vi "Navigation_Main_position_testing may 2.vi"() -> ()   [LabVIEW 2015]
uses:
  <vilib>/myRIO/Instrument Drivers/Onboard IO/PWM/typedefs/PWM Reference.ctl
  <vilib>/myRIO/Common/Instrument Driver Framework/Utilities/typedefs/myRIO Generic Hardware Reference.ctl
  <vilib>/myRIO/Common/Instrument Driver Framework/Utilities/typedefs/Hardware Version Enum.ctl
  <vilib>/myRIO/Common/Instrument Driver Framework/Utilities/typedefs/myRIO v1.0 Reference.ctl
  <vilib>/myRIO/Common/Instrument Driver Framework/Utilities/typedefs/Generic FPGA Reference.ctl
  <vilib>/myRIO/Common/Instrument Driver Framework/myRIO v1.0/PWM/typedefs/PWM Channels Enum.ctl
  <vilib>/myRIO/Instrument Drivers/Onboard IO/PWM/typedefs/PWM Configuration.ctl
  <vilib>/userdefined/High Color/nirio_resource_hc.ctl
  <vilib>/myRIO/Common/Instrument Driver Framework/myRIO v1.0/PWM/vis/myRIO v1.1 Open PWM.vi
  <vilib>/myRIO/Common/Instrument Driver Framework/Utilities/vis/Validate Channels.vi
  <vilib>/myRIO/Common/Instrument Driver Framework/myRIO v1.0/PWM/vis/myRIO v1.0 Reserve PWM.vi
  <vilib>/myRIO/Common/Instrument Driver Framework/myRIO v1.0/PWM/vis/myRIO v1.0 Build MUX Configuration PWM.vi
  <vilib>/myRIO/Common/Instrument Driver Framework/myRIO v1.0/Resource Manager/vis/myRIO v1.0 Reserve Channel List.vi
  <vilib>/myRIO/Common/Instrument Driver Framework/myRIO v1.0/Resource Manager/vis/myRIO v1.0 Create Configuration List.vi
  <vilib>/myRIO/Common/Instrument Driver Framework/myRIO v1.0/Resource Manager/vis/myRIO v1.0 Reserve Channel.vi
  <vilib>/myRIO/Common/Instrument Driver Framework/myRIO v1.0/Resource Manager/vis/myRIO v1.0 Unreserve Channel.vi
  <vilib>/myRIO/Common/Instrument Driver Framework/myRIO v1.0/Resource Manager/vis/myRIO v1.0 Build Mutex Name.vi
  <vilib>/FPGAPlugInAG/myRIO-1900/niLvFpga_Open_myRIO-1900.vi
  <vilib>/rvi/interface/common/dynamic/niFpgaDynamicAddResources.vi
  <vilib>/myRIO/Common/Instrument Driver Framework/Utilities/vis/FPGA Ref Manager.vi
  <vilib>/Utility/error.llb/Error Cluster From Error Code.vi
  <vilib>/myRIO/Common/Instrument Driver Framework/Utilities/vis/Ref Counter.vi
  <vilib>/rvi/errors/niLvFpgaAdjustHostInterfaceError.vi
  <vilib>/Utility/VariantDataType/GetNumericInfo.vi
  <vilib>/myRIO/Common/Instrument Driver Framework/myRIO v1.0/myRIO v1.1 Open.vi
  <vilib>/myRIO/Common/Instrument Driver Framework/Utilities/vis/IO Manager.vi
  <vilib>/myRIO/Common/Instrument Driver Framework/Utilities/vis/Configuration Manager.vi
  <vilib>/myRIO/Common/Instrument Driver Framework/myRIO v1.0/Resource Manager/vis/myRIO v1.0 Configure IO.vi
  <vilib>/myRIO/Common/Instrument Driver Framework/myRIO v1.0/myRIO v1.0 Close.vi
  <vilib>/myRIO/Common/Instrument Driver Framework/myRIO v1.0/PWM/vis/myRIO v1.0 Write PWM.vi
  <vilib>/addons/control/pid/pid.llb/PID (DBL).vi
  <vilib>/rvi/interface/nirviOpenFPGA/nirviOpenFPGA.xnode
  Navi/E/FPGA Bitfiles/NavigationProjec_FPGATarget2_FPGAMainNavigati_PWPHW8gwDxI.lvbitx
  <vilib>/rvi/interface/nirviReadWriteControl/nirviReadWriteControl.xnode
  <vilib>/myRIO/Instrument Drivers/Onboard IO/PWM/vis/myRIO PWM Open.xnode
  <vilib>/myRIO/Instrument Drivers/Onboard IO/PWM/PWM.lvlib
  <vilib>/myRIO/Instrument Drivers/Utilities/Utilities.lvlib
  NiFpgaLv.dll
  <vilib>/rvi/interface/Simulation/niFpgaSimulationCallBeginRW.vi
  <vilib>/addons/control/pid/NI_PID_pid.lvlib
panel:
  out "y1ahead":dbl
  out "angle error":dbl
  out "percent away from x goal":dbl
  out "y desired":dbl
  out "slope desired":dbl
  out "orientation theta desired":dbl
  out "current angle":dbl
  out "current y":dbl
  out "current x":dbl
  out "mining angle":dbl
  out "mining y":dbl
  out "mining x":dbl
  out "mining location":dbl=1.0
  out "distance to goal":dbl
  out "loc_y":dbl
  out "loc_x":dbl
  out "loc_theta":dbl
  in  "motor killswitch":bool
  in  "set start position":bool
  in  "dumping complete":bool
  in  "digging complete?":bool
  in  "position good?":bool
  in  "state":dbl
  in  "case":dbl
  in  "x goal":dbl=9.0
  in  "Encoder Reset":bool
  out "scale":dbl=1.0
  out "reset x y 2":dbl
  out "stop motors":dbl
  out "encoder stop switch":dbl=1.0
  out "left wheels actual pwm":dbl
  out "right wheels actual pwm":dbl
  out "desired pwm right":dbl
  out "desired pwm left":dbl
  out "left setpoint":dbl
  out "right setpoint":dbl
  in  "PID Settings":enum32{"Right PID PWM", "Left PID PWM"}(tab)
  in  "output range right":cluster{"output high":dbl, "output low":dbl}={"output high"=0.13333, "output low"=-0.13333} {"output low" format="%.6f"; "output high" format="%.5f"}
  in  "PID gains right":T1={"proportional gain (Kc)"=0.002, "integral time (Ti, min)"=7e-07, "derivative time (Td, min)"=0.0} {"derivative time (Td, min)" format="%.8f"; "integral time (Ti, min)" format="%.8f"; "proportional gain (Kc)" format="%.8f"}
  out "dt out (s) right":dbl format="%.3f"
  out "PID feedback Right":dbl
  out "Elapsed Time (s) Right":dbl caption="Elapsed Time (s)"
  in  "pid reset right":bool
  in  "output range left":cluster{"output high":dbl, "output low":dbl}={"output high"=0.13333, "output low"=-0.13333} {"output low" format="%.6f"; "output high" format="%.5f"}
  in  "PID gains left":T1={"proportional gain (Kc)"=0.002, "integral time (Ti, min)"=7e-07, "derivative time (Td, min)"=0.0} {"derivative time (Td, min)" format="%.8f"; "integral time (Ti, min)" format="%.8f"; "proportional gain (Kc)" format="%.8f"}
  out "dt out (s) left":dbl format="%.3f"
  out "PID feedback Left":dbl
  out "Elapsed Time (s) Left":dbl caption="Elapsed Time (s)"
  in  "pid reset left":bool
  out "start angle":dbl=1.0
  out "start x":dbl=1.0
  out "start y":dbl
  in  "stuff that i dont want to mess with right now":T2(tab)
  out "RM Linear Velocity (rot/s)":dbl
  out "RR Rot Velocity (rot/s)":dbl
  out "LR Rot Velocity (rot/s)":dbl
  out "LM Rot Velocity (rot/s)":dbl
  out "LF Rot Velocity (rot/s)":dbl
  out "RF Linear Velocity (rot/s)":dbl
  out "Tick Count(mSec) 2":u32 caption="Tick Count(mSec)"
  out "y traveled 2":dbl
  out "x traveled 2":dbl
  out "y position 2":dbl
  out "x position 2":dbl
  out "y dot 2":dbl
  out "distance traveled 2":dbl
  out "psi dot 2":dbl
  out "x dot 2":dbl
  out ".not. x? 2":bool
  out ".not. x? 3":bool
  out "goal reached":bool=TRUE
  out "avg ENC.B":dbl
  out "avg ENC.A":dbl
  out "ENC.B_c.CNTR":i32
  out "ENC.B_b.CNTR":i32
  out "ENC.B_a.CNTR":i32
  out "ENC.A_c.CNTR":i32
  out "ENC.A_b.CNTR":i32
  out "ENC.A_a.CNTR":i32
  out "stage set point parameters":T3(tab)
  out "x straight 1 end":dbl=2.0
  in  "ypstart straight 1":dbl
  in  "ystart":dbl=1.0
  in  "yend straight 1":dbl=2.0
  in  "ypend straight 1":dbl
  out "a straight 1":dbl
  out "b straight 1":dbl
  out "c straight 1":dbl
  out "d straight 1":dbl
  out "x turn end":dbl=7.0
  in  "ystart turn":dbl=1.0
  in  "yend turn":dbl=2.0
  in  "ypstart turn":dbl
  in  "ypend turn":dbl
  out "a turn":dbl
  out "b turn":dbl
  out "c turn":dbl
  out "d turn":dbl
  out "x straight 2 end":dbl=10.0
  in  "yend straight 2":dbl=2.0
  out "a straight 2":dbl
  out "b straight 2":dbl
  out "c straight 2":dbl
  out "d straight 2":dbl
  in  "ypend 2":dbl
  in  "ypstart straight 2":dbl
  in  "mining y 1":dbl=2.0
  in  "mining angle 1":dbl
  in  "mining x 1":dbl=9.0
  in  "mining angle -1":dbl
  in  "mining y -1":dbl=4.0
  in  "mining x -1":dbl=9.0
  out "left pwm":dbl(graph)
  out "right pwm":dbl(graph)
  out "SYS.SELECTA":u8 format="%08b"
  in  "R Min Linear Velocity (ft/s)":dbl=-2.0 format="%#_13g"
  in  "R Max Linear Velocity (ft/s)":dbl=2.0 format="%#_13g"
  in  "L Min Linear Velocity (ft/s)":dbl=-2.0 format="%#_13g"
  in  "L Max Linear Velocity (ft/s)":dbl=2.0 format="%#_13g"
  out "Current Rot Velocity (rot/s)":T4(graph)
  # "Position Information"
  # "move cases along"
  # "end state 0\ngo to state 1"
  # "end state 1\ngo to state 2"
  # "end state 2\ngo to state 3"
  # "end state 3\ngo to state 4"
  # "end state 4\ngo to state 0"
  # "same thing, redundant \nbut can be changed to \nsomething useful later"
  # "this must be true to \ninitialize the routine"
  # "go through the 3\n movement cases"
  # "go through the 3\n movement cases"
  # "Stop Flags \n1=go \n0=stop"
  # "PWM Setpoint"
  # "Initial condtions"
  # "Encoder Values"
  # "Motor Control Parameters"
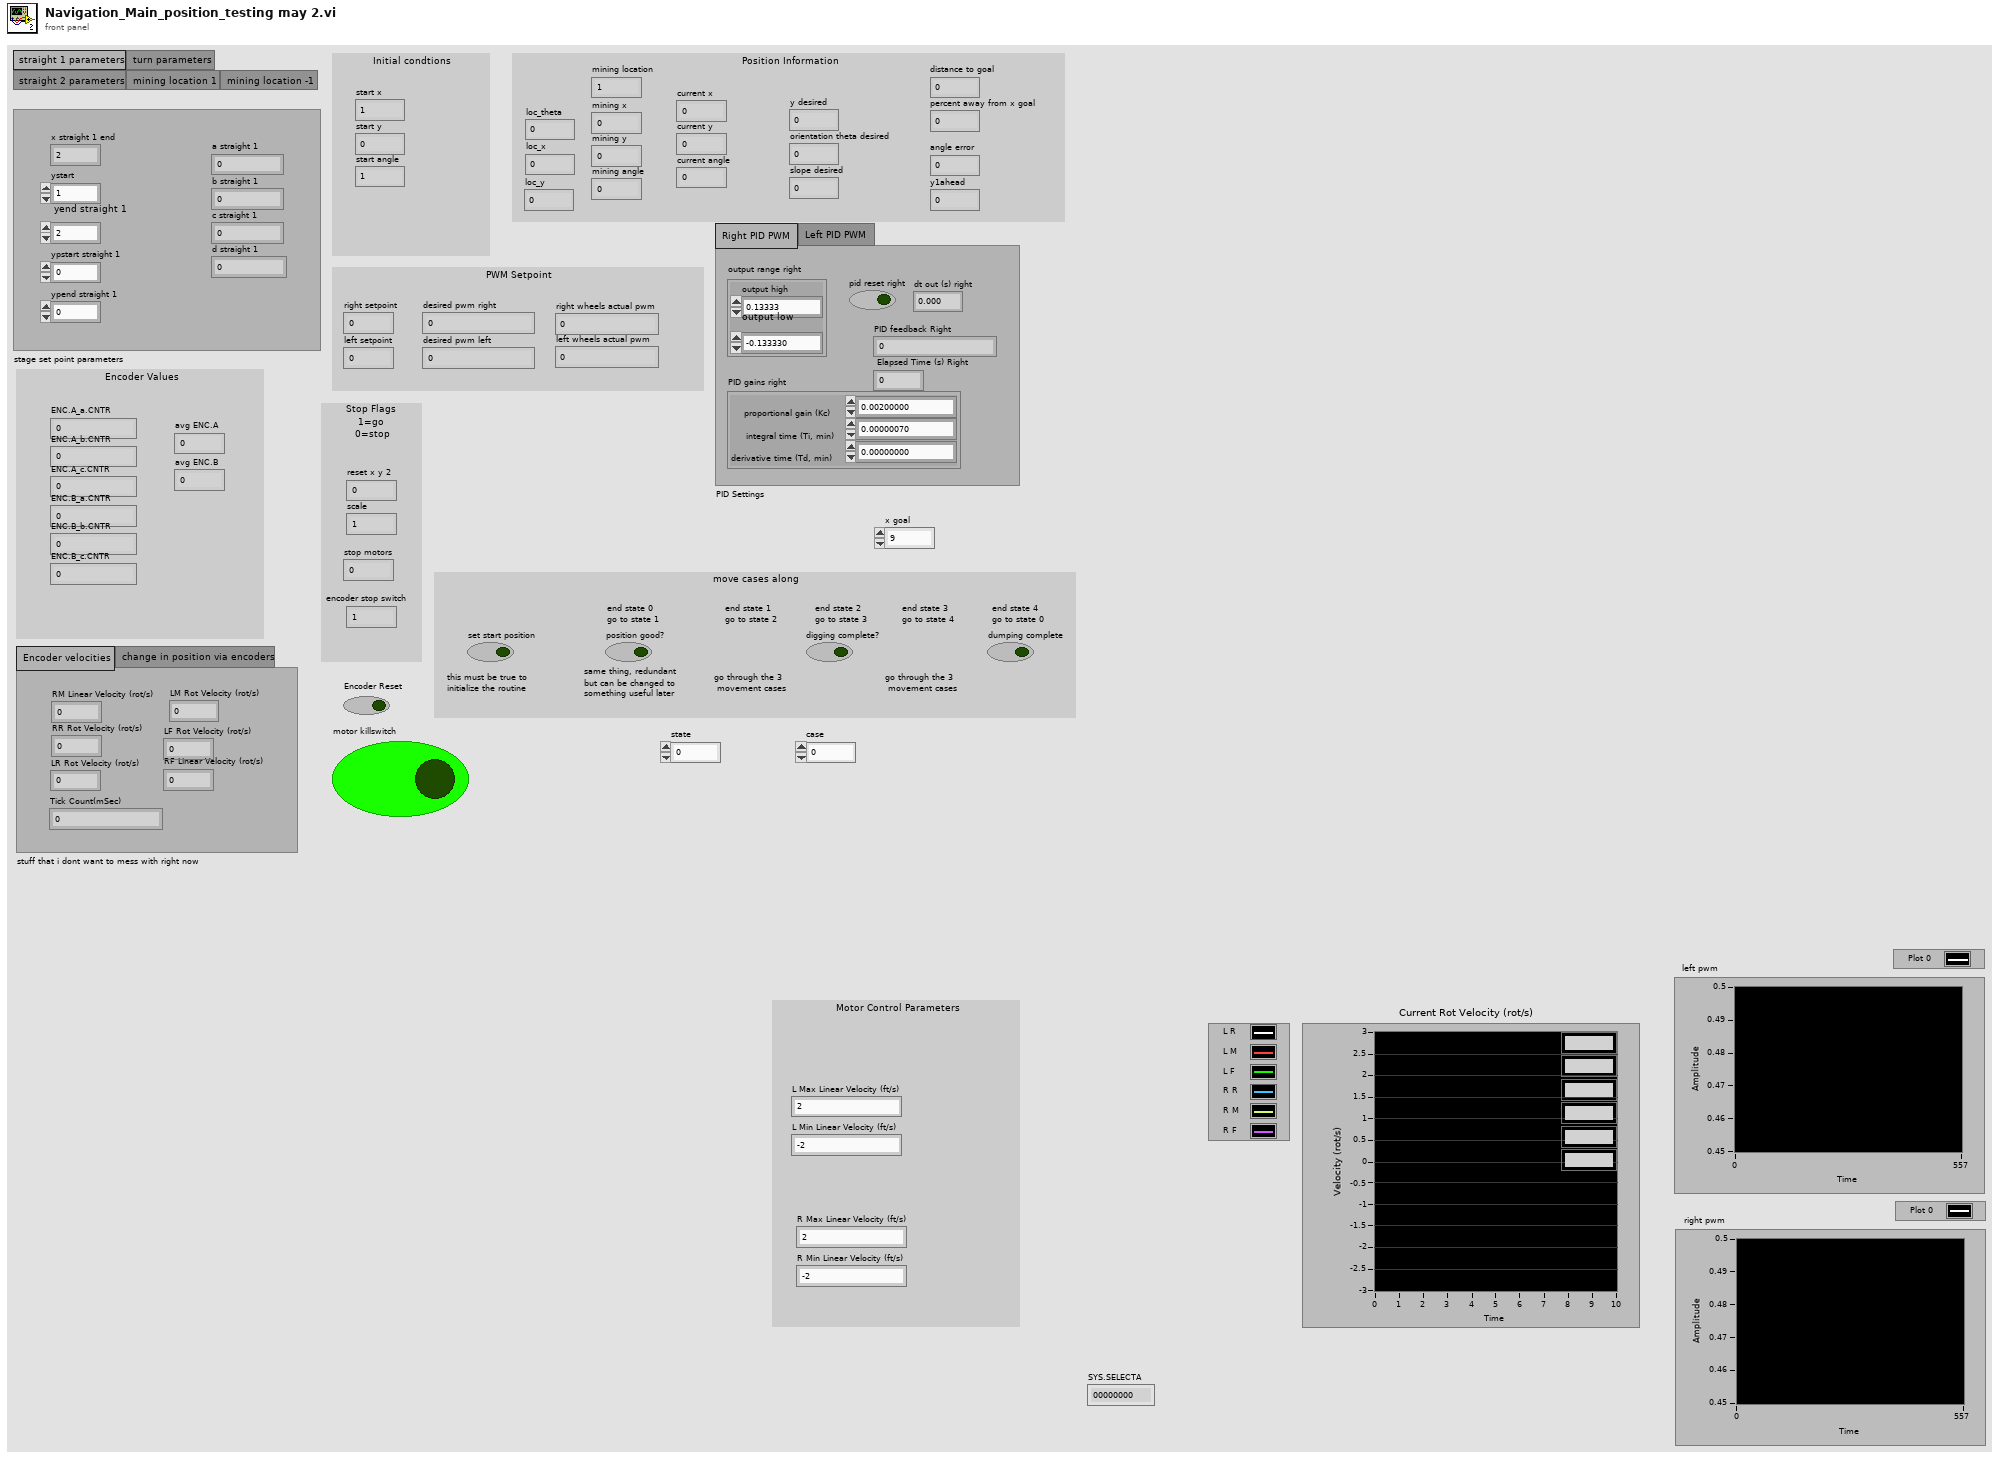
[diagram p1: front panel]
types:
  T1 = cluster{"proportional gain (Kc)":dbl, "integral time (Ti, min)":dbl, "derivative time (Td, min)":dbl}
  T2 = enum32{"Encoder velocities", "change in position via encoders"}
  T3 = enum32{"straight 1 parameters", "turn parameters", "straight 2 parameters", "mining location 1", "mining location -1"}
  T4 = cluster{"Rotational Velocity (RPS)":dbl, "Rotational Velocity (RPS)":dbl, "Rotational Velocity (RPS)":dbl, "Rotational Velocity (RPS)":dbl, "Rotational Velocity (RPS)":dbl, "Rotational Velocity (RPS)":dbl}
  T5 = typedef "nirio_resource_hc.ctl" = tag
  T6 = typedef "Hardware Version Enum.ctl" = enum16{"Unknown", "myRIO-1900", "myRIO-1950", "roboRIO"}
  T7 = typedef "PWM.lvlib/PWM Reference.ctl" = cluster{"myRIO Reference":T8, "PWM Channels Enum":T11, "PWM Configuration":T12}
  T8 = typedef "myRIO Generic Hardware Reference.ctl" = cluster{"myRIO Model":T6, "myRIO Hardware Reference":T9}
  T9 = typedef "myRIO v1.0 Reference.ctl" = cluster{"Generic FPGA Reference":T10, "Allow multiple opens":bool}
  T10 = typedef "Generic FPGA Reference.ctl" = refnum<k20>
  T11 = typedef "PWM Channels Enum.ctl" = enum16{"Not Connected", "C/PWM0", "C/PWM1", "A/PWM0", "A/PWM1", "A/PWM2", "B/PWM0", "B/PWM1", "B/PWM2", "PWM/PWM0", "PWM/PWM1", "PWM/PWM2", "PWM/PWM3", "PWM/PWM4", "PWM/PWM5", "PWM/PWM6", "PWM/PWM7", "PWM/PWM8", "PWM/PWM9"}
  T12 = typedef "PWM.lvlib/PWM Configuration.ctl" = cluster{"Frequency":dbl, "Duty Cycle":dbl}
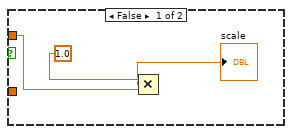
[diagram p3: hidden frame]
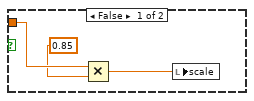
[diagram p4: hidden frame]
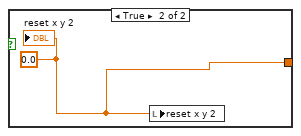
[diagram p5: hidden frame]
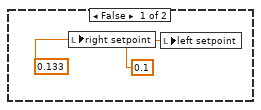
[diagram p6: hidden frame]
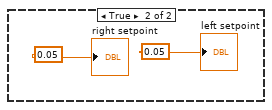
[diagram p7: hidden frame]
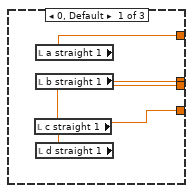
[diagram p8: hidden frame]
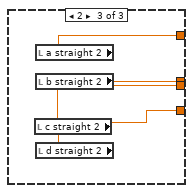
[diagram p9: hidden frame]
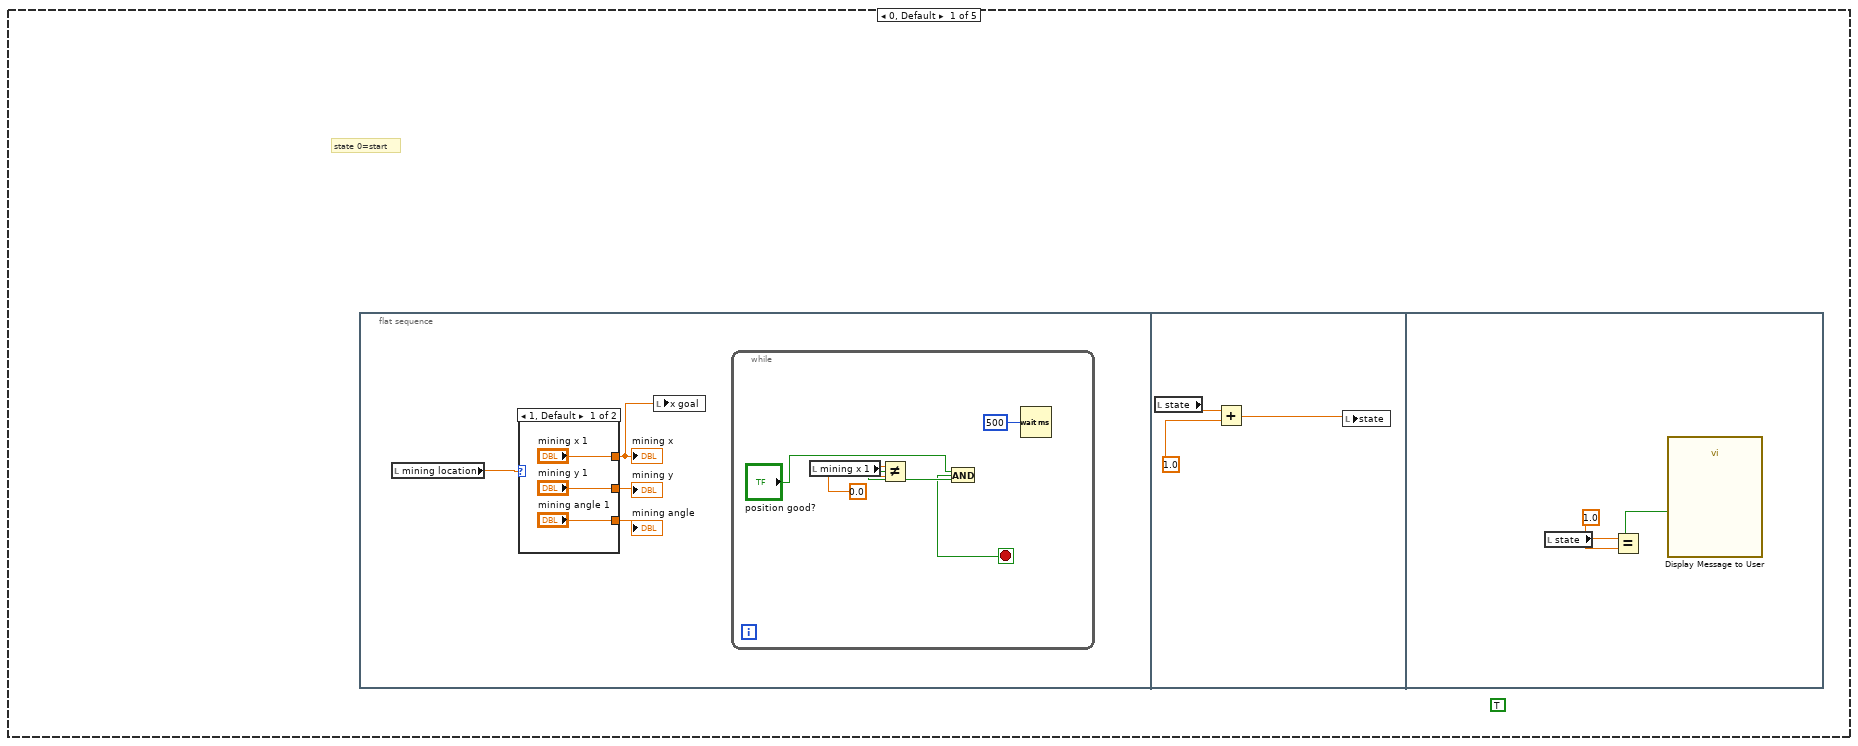
[diagram p10: hidden frame]
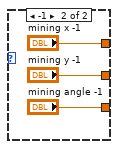
[diagram p11: hidden frame]
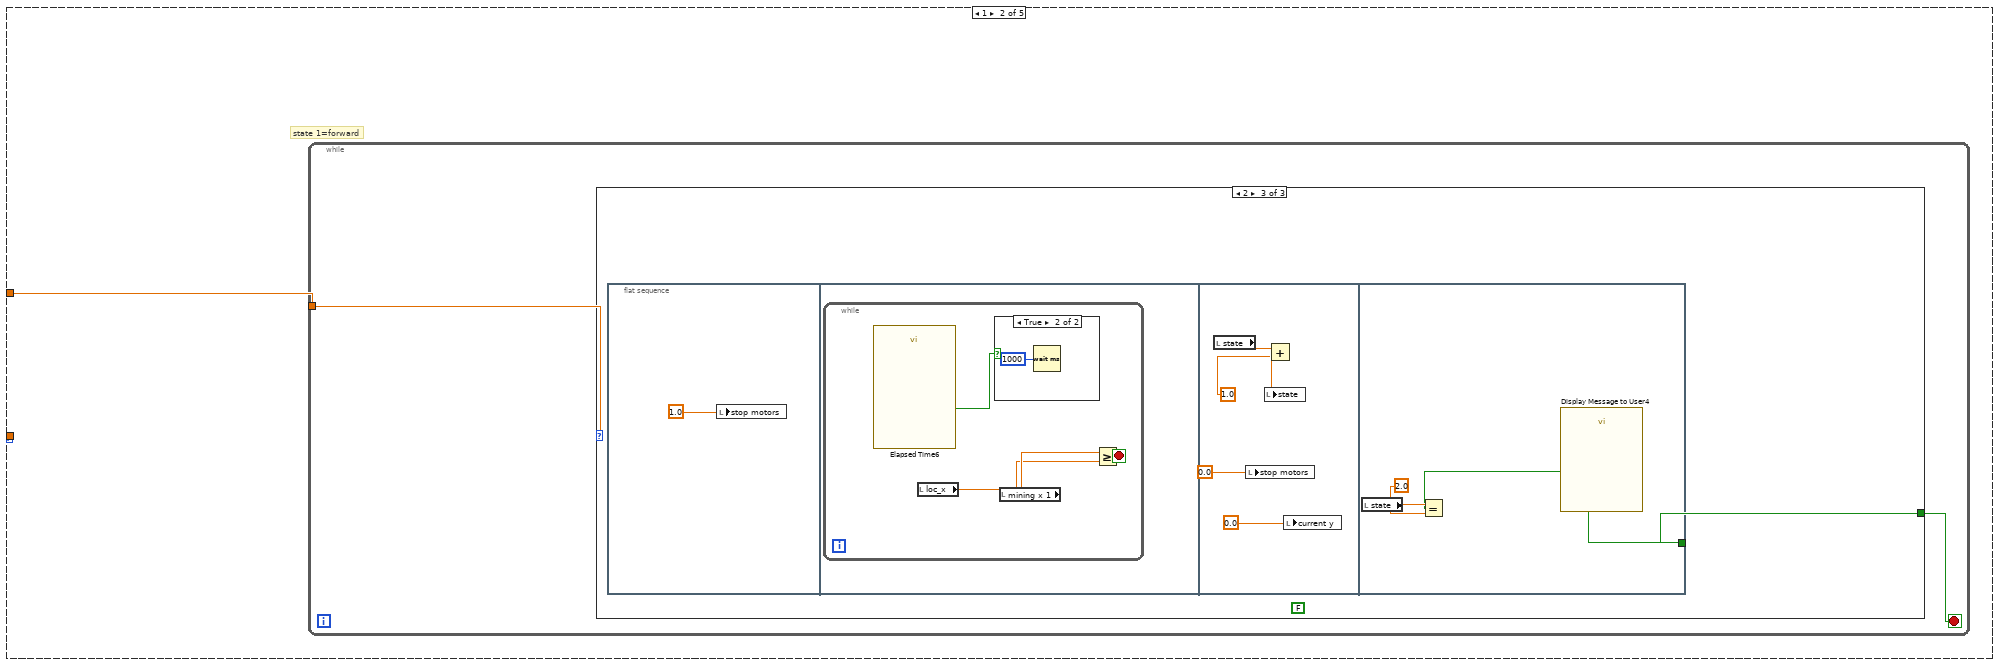
[diagram p12: hidden frame]
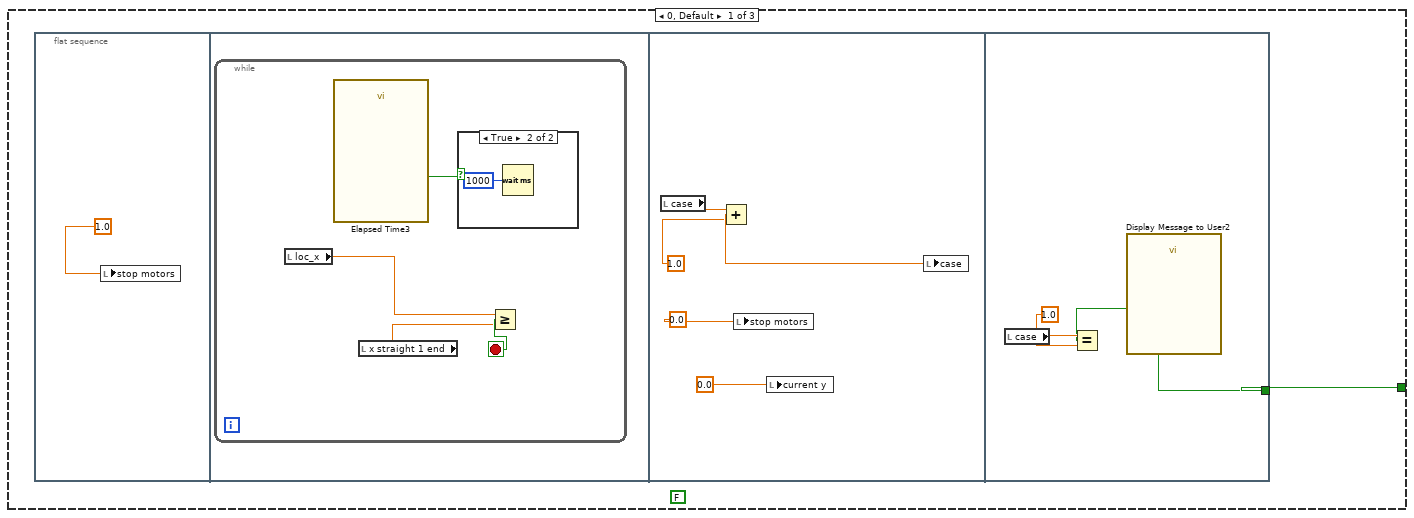
[diagram p13: hidden frame]
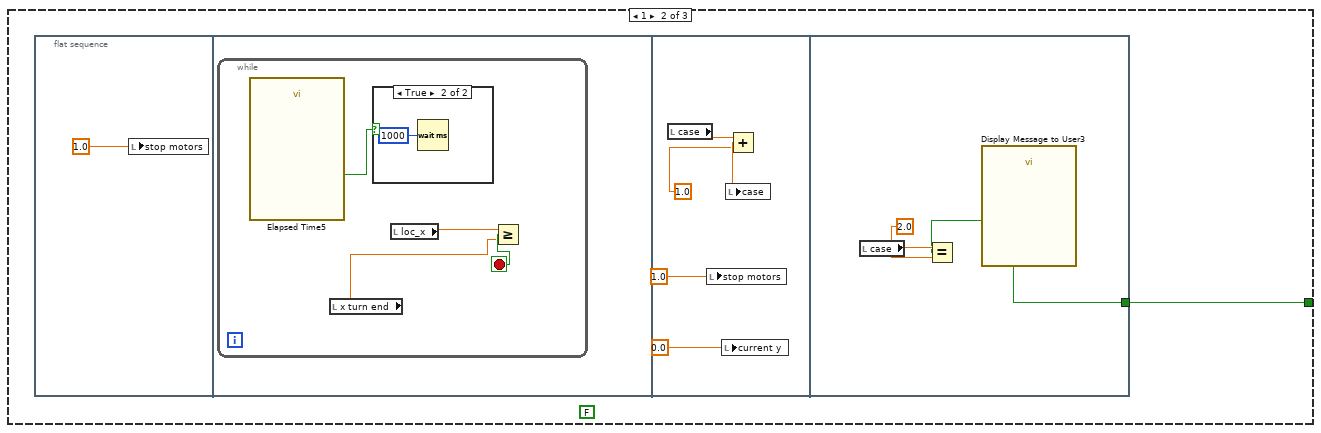
[diagram p15: hidden frame]
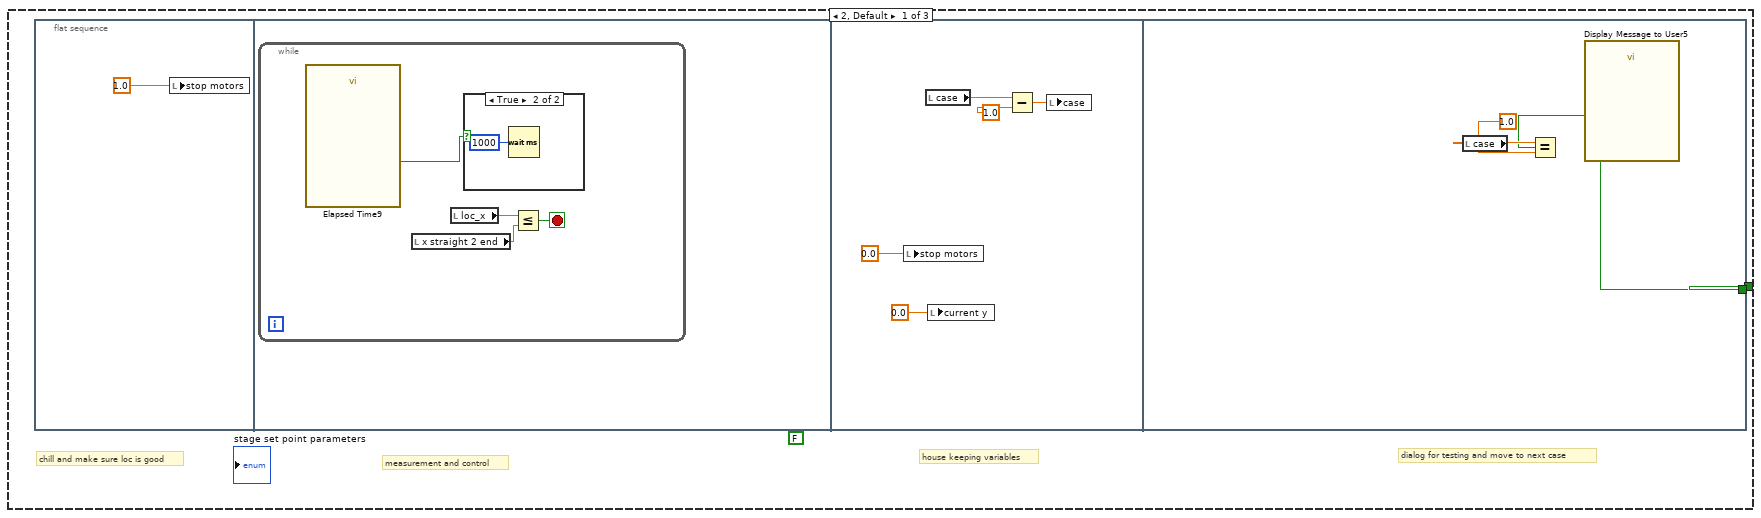
[diagram p18: hidden frame]
diagram:
  n1 = flat-sequence {
    tunnel: [w33] -> w30
    tunnel: [w33] -> w29
    tunnel: [w46] -> w28
    tunnel: [w61] -> w26
    tunnel: [w57] -> w24
    tunnel: [w56] -> w22
    tunnel: [w55] -> w20
    tunnel: [w54] -> w18
    tunnel: [w53] -> w16
    tunnel: ["L Max Linear Velocity (ft/s)"] -> w14
    tunnel: ["L Min Linear Velocity (ft/s)"] -> w12
    tunnel: ["R Max Linear Velocity (ft/s)"] -> w10
    tunnel: ["R Min Linear Velocity (ft/s)"] -> w8
    tunnel: [w48] -> w6
    tunnel: w30 -> [w47]
    tunnel: [w47] -> w4
    tunnel: w29 -> [w48]
    tunnel: [w46] -> w2
    tunnel: w28 -> [w187]
    tunnel: [w187] -> w27
    tunnel: w26 -> [w186]
    tunnel: [w186] -> w25
    tunnel: w24 -> [w185]
    tunnel: [w185] -> w23
    tunnel: w22 -> [w184]
    tunnel: [w184] -> w21
    tunnel: w20 -> [w183]
    tunnel: [w183] -> w19
    tunnel: w18 -> [w182]
    tunnel: [w182] -> w17
    tunnel: w16 -> [w181]
    tunnel: [w181] -> w15
    tunnel: w14 -> [w180]
    tunnel: [w180] -> w13
    tunnel: w12 -> [w179]
    tunnel: [w179] -> w11
    tunnel: w10 -> [w178]
    tunnel: [w178] -> w9
    tunnel: w8 -> [w177]
    tunnel: [w177] -> w7
    tunnel: w6 -> [w176]
    tunnel: [w176] -> w5
    tunnel: w4 -> [w175]
    tunnel: [w175] -> w3
    tunnel: w2 -> [w174]
    tunnel: [w174] -> w1
    tunnel: w27 -> [_]
    tunnel: w25 -> [w196]
    tunnel: w23 -> [w202]
    tunnel: w21 -> [w199]
    tunnel: w19 -> [w198]
    tunnel: w17 -> [w197]
    tunnel: w15 -> [w201]
    tunnel: w13 -> [_]
    tunnel: w11 -> [_]
    tunnel: w9 -> [_]
    tunnel: w7 -> [_]
    tunnel: w5 -> [w204]
    tunnel: w3 -> [w203]
    tunnel: w1 -> [w200]
    frame #0 {
      n2 = flat-sequence {
        tunnel: w34 -> [w39]
        tunnel: [w37] -> w36
        tunnel: w36 -> [w41]
        tunnel: [w41] -> w35
        tunnel: w35 -> [w44]
        tunnel: [w43] -> w33
        frame #0 {
          w38 = u8 32 ("SYS.SELECTA")
          w40 = u8 3 ("ENC.B_c.CNFG")
          n3 = xnode "Read/Write Control"("FPGA VI Reference In"=w39, "ENC.A_a.CNFG"=w40, "ENC.A_b.CNFG"=w40, "ENC.A_c.CNFG"=w40, "ENC.B_a.CNFG"=w40, "ENC.B_b.CNFG"=w40, "ENC.B_c.CNFG"=w40, "SYS.SELECTA"=w38, "SYS.SELECTB"=w38) -> ("FPGA VI Reference Out"=w37:refnum<k20>)  [unwired: 1 in, 1 out]
        }
        frame #1 {
          n4 = Wait (ms)(milliseconds to wait=u32 10) -> ()  [unwired: 1 out]
        }
        frame #2 {
          w45 = u8 1 ("ENC.B_c.CNFG")
          n5 = xnode "Read/Write Control"("FPGA VI Reference In"=w44, "ENC.A_a.CNFG"=w45, "ENC.A_b.CNFG"=w45, "ENC.A_c.CNFG"=w45, "ENC.B_a.CNFG"=w45, "ENC.B_b.CNFG"=w45, "ENC.B_c.CNFG"=w45) -> ("FPGA VI Reference Out"=w43:refnum<k20>)  [unwired: 1 in, 1 out]
        }
      }
      n6 = xnode "Open FPGA VI Reference"("resource name"=tag "RIO0") -> ("FPGA VI Reference Out"=w32:refnum<k20>)  [unwired: 1 in, 1 out]
      n7 = call <vilib>:"Set Custom Bitfile.vi"("Custom FPGA Reference In"=w32) -> ("Custom FPGA Reference Out"=w34:refnum<k20>)  [unwired: 9 in, 1 out]
    }
    frame #1 {
      w58 = 0.5 ("Duty Cycle")
      w46 = 333.333 ("Frequency [Hz]")
      w72 = tag "B/PWM2"  # Right rear ch
      w73 = tag "B/PWM0"  # Right mid ch
      w74 = tag "B/PWM1"  # Right front ch
      w75 = tag "A/PWM2"  # Left rear ch
      w76 = tag "A/PWM1"  # Left mid ch
      w77 = tag "A/PWM0"  # Left front ch
      n8 = xnode "Right  Front"("Channel Name"=w74) -> ("PWM Ref Out"=w68:T7)  [unwired: 2 in, 1 out]
      n9 = xnode "Right  Rear"("Channel Name"=w72) -> ("PWM Ref Out"=w66:T7)  [unwired: 2 in, 1 out]
      n10 = xnode "Left Front"("Channel Name"=w77) -> ("PWM Ref Out"=w71:T7)  [unwired: 2 in, 1 out]
      n11 = xnode "Right  Mid"("Channel Name"=w73) -> ("PWM Ref Out"=w67:T7)  [unwired: 2 in, 1 out]
      n12 = xnode "Left Rear"("Channel Name"=w75) -> ("PWM Ref Out"=w69:T7)  [unwired: 2 in, 1 out]
      n13 = xnode "Left Mid"("Channel Name"=w76) -> ("PWM Ref Out"=w70:T7)  [unwired: 2 in, 1 out]
      n14 = call <vilib>:"Set Frequency.vi"("Frequency [Hz]"=w46, "PWM Ref In"=w68) -> ("PWM Ref Out"=w62:T7)  [unwired: 7 in, 1 out]
      n15 = call <vilib>:"Set Frequency.vi"("Frequency [Hz]"=w46, "PWM Ref In"=w67) -> ("PWM Ref Out"=w63:T7)  [unwired: 7 in, 1 out]
      n16 = call <vilib>:"Set Frequency.vi"("Frequency [Hz]"=w46, "PWM Ref In"=w66) -> ("PWM Ref Out"=w64:T7)  [unwired: 7 in, 1 out]
      n17 = call <vilib>:"Set Frequency.vi"("Frequency [Hz]"=w46, "PWM Ref In"=w70) -> ("PWM Ref Out"=w59:T7)  [unwired: 7 in, 1 out]
      n18 = call <vilib>:"Set Frequency.vi"("Frequency [Hz]"=w46, "PWM Ref In"=w71) -> ("PWM Ref Out"=w65:T7)  [unwired: 7 in, 1 out]
      n19 = call <vilib>:"Set Frequency.vi"("Frequency [Hz]"=w46, "PWM Ref In"=w69) -> ("PWM Ref Out"=w60:T7)  [unwired: 7 in, 1 out]
      n20 = call <vilib>:"Set Duty Cycle.vi"("Duty Cycle"=w58, "PWM Ref In"=w62) -> ("PWM Ref Out"=w57:T7)  [unwired: 7 in, 1 out]
      n21 = call <vilib>:"Set Duty Cycle.vi"("Duty Cycle"=w58, "PWM Ref In"=w63) -> ("PWM Ref Out"=w56:T7)  [unwired: 7 in, 1 out]
      n22 = call <vilib>:"Set Duty Cycle.vi"("Duty Cycle"=w58, "PWM Ref In"=w64) -> ("PWM Ref Out"=w55:T7)  [unwired: 7 in, 1 out]
      n23 = call <vilib>:"Set Duty Cycle.vi"("Duty Cycle"=w58, "PWM Ref In"=w59) -> ("PWM Ref Out"=w54:T7)  [unwired: 7 in, 1 out]
      n24 = call <vilib>:"Set Duty Cycle.vi"("Duty Cycle"=w58, "PWM Ref In"=w65) -> ("PWM Ref Out"=w53:T7)  [unwired: 7 in, 1 out]
      n25 = call <vilib>:"Set Duty Cycle.vi"("Duty Cycle"=w58, "PWM Ref In"=w60) -> ("PWM Ref Out"=w61:T7)  [unwired: 7 in, 1 out]
    }
    frame #2 {
      n26 = while {
        stop <- w188 stop-if-true
        n27 = case shown="True" "set start position" {
          selector: "set start position" -> [_ w195]
          tunnel: [_ w195] -> w188
          frame False {
          }
          frame True {
            n28 = shared-variable "RT myRIO Target - Overlord\\Localization_Variables_r0.lvlib\\loc_x"() -> (→"start x":dbl)  [unwired: 1 in, 1 out]
            n29 = shared-variable "RT myRIO Target - Overlord\\Localization_Variables_r0.lvlib\\loc_y"() -> (→"start y":dbl)  [unwired: 1 in, 1 out]
            n30 = shared-variable "RT myRIO Target - Overlord\\Localization_Variables_r0.lvlib\\loc_theta"() -> (→"start angle":dbl)  [unwired: 1 in, 1 out]
            n31 = Wait (ms)(milliseconds to wait=u32 500) -> ()  [unwired: 1 out]
            "stop motors" <- 1.0 ("stop motors")
          }
        }
      }
    }
    frame #3 {
      (unwired) FALSE
      # "Uses quadrature encoder tick count to calculate rotational and linear velocity for a wheel."
      # "20ms loop delay to allow the encoder to travel far enough for a good update. 20ms provides 50Hz update rate to match motor PWM output rate."
      n32 = flat-sequence {
        frame #0 {
          # "this calculates from the \nmeasured start to the desired end"
          n33 = local read "x straight 1 end"() -> (w274:dbl)
          n34 = local read "start x"() -> (w275:dbl)
          n35 = call "path coefs.vi"("ypend"="ypend straight 1", "ypstart"="ypstart straight 1", "yend"="yend straight 1", "ystart"="ystart", "xend"=w274, "xstart"=w275) -> ("d"=→"d straight 1":dbl, "c"=→"c straight 1":dbl, "b"=→"b straight 1":dbl, "a"=→"a straight 1":dbl)  [unwired: 2 in]
        }
        frame #1 {
          # "right now this measures from the\ndesired start to the desired end"
          n36 = local read "x straight 1 end"() -> (w292:dbl)
          n37 = local read "x turn end"() -> (w293:dbl)
          n38 = call "path coefs.vi"("ypend"="ypend turn", "ypstart"="ypstart turn", "yend"="yend turn", "ystart"="ystart turn", "xend"=w293, "xstart"=w292) -> ("d"=→"d turn":dbl, "c"=→"c turn":dbl, "b"=→"b turn":dbl, "a"=→"a turn":dbl)  [unwired: 2 in]
        }
        frame #2 {
          # "right now this measures from \nthe desired start to the desired end"
          n39 = local read "x straight 2 end"() -> (w303:dbl)
          n40 = local read "x turn end"() -> (w302:dbl)
          n41 = local read "yend turn"() -> (w294:dbl)
          n42 = call "path coefs.vi"("ypend"="ypend 2", "ypstart"="ypstart straight 2", "yend"="yend straight 2", "ystart"=w294, "xend"=w303, "xstart"=w302) -> ("d"=→"d straight 2":dbl, "c"=→"c straight 2":dbl, "b"=→"b straight 2":dbl, "a"=→"a straight 2":dbl)  [unwired: 2 in]
        }
      }
      n43 = while {
        stop <- w306 stop-if-true
        n44 = case shown="3" "state" {
          tunnel: [_ _ _ _ w441] -> w306
          tunnel: "case" -> [_ w329 w380 _ _]
          tunnel: "state" -> [_ _ _ _ _]
          frame 0, Default {
            (unwired) TRUE
            # "state 0=start"
            n45 = flat-sequence {
              frame #0 {
                n46 = local read "mining location"() -> (w310:dbl)
                n47 = case shown="1, Default" w310 {
                  tunnel: ["mining x 1" "mining x -1"] -> w307
                  tunnel: ["mining y 1" "mining y -1"] -> w309
                  tunnel: ["mining angle 1" "mining angle -1"] -> w308
                  frame 1, Default {
                  }
                  frame -1 {
                  }
                }
                "mining x" <- w307
                "mining y" <- w309
                "mining angle" <- w308
                n48 = local write "x goal"(w307) -> ()
                n49 = while {
                  stop <- w317 stop-if-true
                  n50 = local read "mining x 1"() -> (w322:dbl)
                  n51 = Not Equal?(x=w322, y=0.0) -> (x != y?=w318:bool)
                  n52 = And(x="position good?", y=w318) -> (x .and. y?=w317:bool)
                  n53 = Wait (ms)(milliseconds to wait=u32 500) -> ()  [unwired: 1 out]
                }
              }
              frame #1 {
                n54 = local read "state"() -> (w323:dbl)
                n55 = Add(x=w323, y=1.0) -> (x+y=w325:dbl)
                n56 = local write "state"(w325) -> ()
              }
              frame #2 {
                n57 = local read "state"() -> (w328:dbl)
                n58 = Equal?(x=w328, y=1.0) -> (x = y?=w326:bool)
                n59 = call "Display Message to User"("Enable"=w326) -> ()  [unwired: 9 in, 2 out]
              }
            }
          }
          frame 1 {
            # "state 1=forward"
            n60 = while {
              tunnel: w329 -> [w330]
              stop <- w331 stop-if-true
              n61 = case shown="2" w330 {
                tunnel: [w332 w348 w364] -> w331
                frame 0, Default {
                  (unwired) FALSE
                  n62 = flat-sequence {
                    tunnel: [w344] -> w332
                    frame #0 {
                      n63 = local write "stop motors"(1.0) -> ()
                    }
                    frame #1 {
                      n64 = while {
                        stop <- w337 stop-if-true
                        n65 = local read "loc_x"() -> (w336:dbl)
                        n66 = call "Elapsed Time3"() -> ("Time has Elapsed"=w334:bool)  [unwired: 12 in, 7 out]
                        n67 = local read "x straight 1 end"() -> (w335:dbl)
                        n68 = case shown="True" w334 {
                          frame False {
                          }
                          frame True {
                            n69 = Wait (ms)(milliseconds to wait=u32 1000) -> ()  [unwired: 1 out]
                          }
                        }
                        n70 = Greater Or Equal?(x=w336, y=w335) -> (x >= y?=w337:bool)
                      }
                    }
                    frame #2 {
                      n71 = local read "case"() -> (w341:dbl)
                      n72 = Add(x=w341, y=1.0) -> (x+y=w343:dbl)
                      n73 = local write "stop motors"(0.0) -> ()
                      n74 = local write "current y"(0.0) -> ()
                      n75 = local write "case"(w343) -> ()
                    }
                    frame #3 {
                      n76 = local read "case"() -> (w347:dbl)
                      n77 = Equal?(x=w347, y=1.0) -> (x = y?=w345:bool)
                      n78 = call "Display Message to User2"("Enable"=w345) -> ("OK"=w344:bool)  [unwired: 9 in, 1 out]
                    }
                  }
                }
                frame 1 {
                  (unwired) FALSE
                  n79 = flat-sequence {
                    tunnel: [w360] -> w348
                    frame #0 {
                      n80 = local write "stop motors"(1.0) -> ()
                    }
                    frame #1 {
                      n81 = while {
                        stop <- w353 stop-if-true
                        n82 = call "Elapsed Time5"() -> ("Time has Elapsed"=w350:bool)  [unwired: 12 in, 7 out]
                        n83 = local read "x turn end"() -> (w351:dbl)
                        n84 = case shown="True" w350 {
                          frame False {
                          }
                          frame True {
                            n85 = Wait (ms)(milliseconds to wait=u32 1000) -> ()  [unwired: 1 out]
                          }
                        }
                        n86 = local read "loc_x"() -> (w352:dbl)
                        n87 = Greater Or Equal?(x=w352, y=w351) -> (x >= y?=w353:bool)
                      }
                    }
                    frame #2 {
                      n88 = local read "case"() -> (w357:dbl)
                      n89 = local write "stop motors"(1.0) -> ()
                      n90 = local write "current y"(0.0) -> ()
                      n91 = Add(x=w357, y=1.0) -> (x+y=w359:dbl)
                      n92 = local write "case"(w359) -> ()
                    }
                    frame #3 {
                      n93 = local read "case"() -> (w363:dbl)
                      n94 = Equal?(x=w363, y=2.0) -> (x = y?=w361:bool)
                      n95 = call "Display Message to User3"("Enable"=w361) -> ("OK"=w360:bool)  [unwired: 9 in, 1 out]
                    }
                  }
                }
                frame 2 {
                  (unwired) FALSE
                  n96 = flat-sequence {
                    tunnel: [w376] -> w364
                    frame #0 {
                      n97 = local write "stop motors"(1.0) -> ()
                    }
                    frame #1 {
                      n98 = while {
                        stop <- w369 stop-if-true
                        n99 = call "Elapsed Time6"() -> ("Time has Elapsed"=w366:bool)  [unwired: 12 in, 7 out]
                        n100 = local read "loc_x"() -> (w368:dbl)
                        n101 = case shown="True" w366 {
                          frame False {
                          }
                          frame True {
                            n102 = Wait (ms)(milliseconds to wait=u32 1000) -> ()  [unwired: 1 out]
                          }
                        }
                        n103 = local read "mining x 1"() -> (w367:dbl)
                        n104 = Greater Or Equal?(x=w368, y=w367) -> (x >= y?=w369:bool)
                      }
                    }
                    frame #2 {
                      n105 = local read "state"() -> (w373:dbl)
                      n106 = local write "stop motors"(0.0) -> ()
                      n107 = Add(x=w373, y=1.0) -> (x+y=w375:dbl)
                      n108 = local write "state"(w375) -> ()
                      n109 = local write "current y"(0.0) -> ()
                    }
                    frame #3 {
                      n110 = local read "state"() -> (w379:dbl)
                      n111 = Equal?(x=w379, y=2.0) -> (x = y?=w377:bool)
                      n112 = call "Display Message to User4"("Enable"=w377) -> ("OK"=w376:bool)  [unwired: 9 in, 1 out]
                    }
                  }
                }
              }
            }
          }
          frame 3 {
            # "state 3=return"
            n113 = while {
              tunnel: w380 -> [w381]
              stop <- w382 stop-if-true
              n114 = case shown="1" w381 {
                tunnel: [w383 w399 w415] -> w382
                frame 2, Default {
                  (unwired) FALSE
                  # "dialog for testing and move to next case"
                  # "measurement and control"
                  # "chill and make sure loc is good"
                  # "house keeping variables"
                  n115 = flat-sequence {
                    tunnel: [w395] -> w383
                    frame #0 {
                      n116 = local write "stop motors"(1.0) -> ()
                    }
                    frame #1 {
                      n117 = while {
                        stop <- w388 stop-if-true
                        n118 = call "Elapsed Time9"() -> ("Time has Elapsed"=w385:bool)  [unwired: 12 in, 7 out]
                        n119 = local read "x straight 2 end"() -> (w386:dbl)
                        n120 = local read "loc_x"() -> (w387:dbl)
                        n121 = case shown="True" w385 {
                          frame False {
                          }
                          frame True {
                            n122 = Wait (ms)(milliseconds to wait=u32 1000) -> ()  [unwired: 1 out]
                          }
                        }
                        n123 = Less Or Equal?(x=w387, y=w386) -> (x <= y?=w388:bool)
                      }
                    }
                    frame #2 {
                      n124 = local write "stop motors"(0.0) -> ()
                      n125 = local read "case"() -> (w392:dbl)
                      n126 = local write "current y"(0.0) -> ()
                      n127 = Subtract(x=w392, y=1.0) -> (x-y=w394:dbl)
                      n128 = local write "case"(w394) -> ()
                    }
                    frame #3 {
                      n129 = local read "case"() -> (w398:dbl)
                      n130 = Equal?(x=w398, y=1.0) -> (x = y?=w396:bool)
                      n131 = call "Display Message to User5"("Enable"=w396) -> ("OK"=w395:bool)  [unwired: 9 in, 1 out]
                    }
                  }
                }
                frame 1 {
                  (unwired) FALSE
                  n132 = flat-sequence {
                    tunnel: [w411] -> w399
                    frame #0 {
                      n133 = local write "stop motors"(1.0) -> ()
                    }
                    frame #1 {
                      n134 = while {
                        stop <- w404 stop-if-true
                        n135 = call "Elapsed Time8"() -> ("Time has Elapsed"=w401:bool)  [unwired: 12 in, 7 out]
                        n136 = local read "x turn end"() -> (w402:dbl)
                        n137 = local read "current x"() -> (w403:dbl)
                        n138 = case shown="True" w401 {
                          frame False {
                          }
                          frame True {
                            n139 = Wait (ms)(milliseconds to wait=u32 1000) -> ()  [unwired: 1 out]
                          }
                        }
                        n140 = Less Or Equal?(x=w403, y=w402) -> (x <= y?=w404:bool)
                      }
                    }
                    frame #2 {
                      n141 = local read "case"() -> (w409:dbl)
                      n142 = local write "stop motors"(0.0) -> ()
                      n143 = local write "current y"(0.0) -> ()
                      n144 = Subtract(x=w409, y=1.0) -> (x-y=w408:dbl)
                      n145 = local write "case"(w408) -> ()
                    }
                    frame #3 {
                      n146 = local read "case"() -> (w414:dbl)
                      n147 = Equal?(x=w414, y=0.0) -> (x = y?=w412:bool)
                      n148 = call "Display Message to User6"("Enable"=w412) -> ("OK"=w411:bool)  [unwired: 9 in, 1 out]
                    }
                  }
                }
                frame 0 {
                  (unwired) FALSE
                  n149 = flat-sequence {
                    tunnel: [w427] -> w415
                    frame #0 {
                      n150 = local write "stop motors"(1.0) -> ()
                    }
                    frame #1 {
                      n151 = while {
                        stop <- w420 stop-if-true
                        n152 = call "Elapsed Time7"() -> ("Time has Elapsed"=w417:bool)  [unwired: 12 in, 7 out]
                        n153 = local read "x straight 1 end"() -> (w418:dbl)
                        n154 = case shown="True" w417 {
                          frame False {
                          }
                          frame True {
                            n155 = Wait (ms)(milliseconds to wait=u32 1000) -> ()  [unwired: 1 out]
                          }
                        }
                        n156 = local read "loc_x"() -> (w419:dbl)
                        n157 = Less Or Equal?(x=w419, y=w418) -> (x <= y?=w420:bool)
                      }
                    }
                    frame #2 {
                      n158 = local read "state"() -> (w424:dbl)
                      n159 = local write "stop motors"(0.0) -> ()
                      n160 = Add(x=w424, y=1.0) -> (x+y=w426:dbl)
                      n161 = local write "state"(w426) -> ()
                      n162 = local write "current y"(0.0) -> ()
                    }
                    frame #3 {
                      n163 = local read "state"() -> (w430:dbl)
                      n164 = Equal?(x=w430, y=4.0) -> (x = y?=w428:bool)
                      n165 = call "Display Message to User7"("Enable"=w428) -> ("OK"=w427:bool)  [unwired: 9 in, 1 out]
                    }
                  }
                }
              }
            }
          }
          frame 2 {
            # "state 2=dig"
            n166 = while {
              stop <- w431 stop-if-true
              (unwired) FALSE
              n167 = flat-sequence {
                tunnel: [w437] -> w431
                frame #0 {
                  n168 = while {
                    stop <- "digging complete?" stop-if-true
                  }
                }
                frame #1 {
                  n169 = local read "state"() -> (w435:dbl)
                  n170 = local read "start x"() -> (w433:dbl)
                  n171 = Add(x=w435, y=1.0) -> (x+y=w434:dbl)
                  n172 = local write "state"(w434) -> ()
                  n173 = local write "x goal"(w433) -> ()
                }
                frame #2 {
                  n174 = local read "state"() -> (w440:dbl)
                  n175 = Equal?(x=w440, y=3.0) -> (x = y?=w438:bool)
                  n176 = call "Display Message to User8"("Enable"=w438) -> ("OK"=w437:bool)  [unwired: 9 in, 1 out]
                }
              }
            }
          }
          frame 4 {
            (unwired) FALSE
            # "state 4=dump"
            n177 = flat-sequence {
              tunnel: [w447] -> w441
              frame #0 {
                n178 = while {
                  stop <- "dumping complete" stop-if-true
                }
              }
              frame #1 {
                n179 = local read "mining location"() -> (w445:dbl)
                n180 = local write "state"(0.0) -> ()
                n181 = Multiply(x=w445, y=-1.0) -> (x*y=w443:dbl)
                n182 = local write "mining location"(w443) -> ()
              }
              frame #2 {
                n183 = local read "state"() -> (w450:dbl)
                n184 = Equal?(x=w450, y=3.0) -> (x = y?=w448:bool)
                n185 = call "Display Message to User9"("Enable"=w448) -> ("OK"=w447:bool)  [unwired: 9 in, 1 out]
              }
            }
          }
        }
      }
      n186 = while {
        stop <- FALSE stop-if-true
        n187 = local read "case"() -> (w256:dbl)
        n188 = case shown="1" w256 {
          tunnel: [w265 w269 w273] -> w260
          tunnel: [w264 w268 w272] -> w259
          tunnel: [w263 w267 w271] -> w258
          tunnel: [w262 w266 w270] -> w257
          frame 0, Default {
            n189 = local read "c straight 1"() -> (w263:dbl)
            n190 = local read "a straight 1"() -> (w265:dbl)
            n191 = local read "b straight 1"() -> (w264:dbl)
            n192 = local read "d straight 1"() -> (w262:dbl)
          }
          frame 1 {
            n193 = local read "c turn"() -> (w267:dbl)
            n194 = local read "a turn"() -> (w269:dbl)
            n195 = local read "b turn"() -> (w268:dbl)
            n196 = local read "d turn"() -> (w266:dbl)
          }
          frame 2 {
            n197 = local read "c straight 2"() -> (w271:dbl)
            n198 = local read "a straight 2"() -> (w273:dbl)
            n199 = local read "b straight 2"() -> (w272:dbl)
            n200 = local read "d straight 2"() -> (w270:dbl)
          }
        }
        n201 = local read "current x"() -> (w255:dbl)
        n202 = formula code="yshould=(a*x**3)/3+(b*x**2)/3+(c*x)/3+d/3;\ny1ahead=(a*(x+1)**3)/3+(b*(x+1)**2)/3+(c*(x+1))/3+d/3;\nslope=(a*x**2 + (2*b*x)/3 + c/3);\nrobot_orientation_theta=(atan(slope));\nleftwheel_x=(-1*sin(robot_orientation_theta)+x);\nrightwheel_x=(1*sin(robot_orientation_theta)+x);\nleftwheel_y=(1*cos(robot_orientation_theta)+yshould);\nrightwheel_y=(-1*cos(robot_orientation_theta)+yshould);"("a"=w260, "b"=w259, "c"=w258, "d"=w257, "x"=w255) -> ("yshould"=→"y desired":dbl, "slope"=→"slope desired":dbl, "robot_orientation_theta"=w252:dbl, "y1ahead"=→"y1ahead":dbl)  [unwired: 4 out]
        "orientation theta desired" <- w252
        n203 = local read "current angle"() -> (w251:dbl)
        n204 = Subtract(x=w252, y=w251) -> (x-y=→"angle error":dbl)
      }
      n205 = while {
        shift-right: [w499] -> _
        shift-left: _ -> [w537]
        shift-right: [w496] -> _
        shift-left: _ -> [w536]
        shift-right: [w498] -> _
        shift-left: _ -> [w511]
        shift-right: [w497] -> _
        shift-left: _ -> [w510]
        stop <- FALSE stop-if-true
        w532 = 28.0  # width wheel to wheel
        w533 = 4.0  # wheel radius
        n206 = local read "ENC.B_a.CNTR"() -> (w542:i32)
        n207 = local read "ENC.B_b.CNTR"() -> (w541:i32)
        n208 = local read "ENC.A_a.CNTR"() -> (w545:i32)
        n209 = local read "ENC.A_b.CNTR"() -> (w544:i32)
        n210 = local read "ENC.A_c.CNTR"() -> (w543:i32)
        n211 = local read "ENC.B_c.CNTR"() -> (w540:i32)
        n212 = local read "reset x y 2"() -> (w495:dbl)
        n213 = Compound Arithmetic op=ADD(w542, w541, w540) -> (w548:i32)
        n214 = Compound Arithmetic op=ADD(w545, w544, w543) -> (w549:i32)
        n215 = Multiply(x=w495, y=w510) -> (x*y=w501:dbl)
        n216 = Multiply(x=w495, y=w511) -> (x*y=w502:dbl)
        n217 = Multiply(x=w495, y=w536) -> (x*y=w500:dbl)
        n218 = Multiply(x=w495, y=w537) -> (x*y=w503:dbl)
        n219 = Divide(x=w548, y=3) -> (x/y=w535:dbl)
        "avg ENC.B" <- w535
        n220 = Divide(x=w549, y=3) -> (x/y=w538:dbl)
        "avg ENC.A" <- w538
        n221 = Subtract(x=w535, y=w500) -> (x-y=w525:dbl)
        n222 = Subtract(x=w538, y=w503) -> (x-y=w526:dbl)
        n223 = Divide(x=w533, y=w532) -> (x/y=w528:dbl)
        n224 = Add(x=w526, y=w525) -> (x+y=w530:dbl)
        n225 = Square(x=w526) -> (x^2=w523:dbl)
        n226 = Square(x=w525) -> (x^2=w524:dbl)
        n227 = Subtract(x=w526, y=w525) -> (x-y=w529:dbl)
        n228 = Divide(x=w533, y=2.0) -> (x/y=w531:dbl)
        n229 = Multiply(x=w529, y=w528) -> (x*y=→"psi dot 2":dbl)
        n230 = Multiply(x=w530, y=w531) -> (x*y=w519:dbl)
        n231 = Add(x=w523, y=w524) -> (x+y=w522:dbl)
        n232 = Inverse Tangent(1:w529) -> (0:w527:dbl)
        n233 = Cosine(x=w527) -> (cos(x)=w520:dbl)
        n234 = Sine(x=w527) -> (sin(x)=w521:dbl)
        n235 = Multiply(x=w519, y=w520) -> (x*y=w517:dbl)
        "x dot 2" <- w517
        n236 = Multiply(x=w519, y=w521) -> (x*y=w518:dbl)
        "y dot 2" <- w518
        n237 = Square Root(x=w522) -> (sqrt(x)=w516:dbl)
        n238 = local read "reset x y 2"() -> (w493:dbl)
        n239 = Multiply(x=w516, y=w493) -> (x*y=w494:dbl)
        "distance traveled 2" <- w494
        n240 = Multiply(x=w494, y=w517) -> (x*y=w515:dbl)
        "x traveled 2" <- w515
        n241 = Multiply(x=w494, y=w518) -> (x*y=w514:dbl)
        "y traveled 2" <- w514
        n242 = Add(x=w501, y=w515) -> (x+y=w513:dbl)
        n243 = Add(x=w502, y=w514) -> (x+y=w505:dbl)
        n244 = Multiply(x=w538, y=w493) -> (x*y=w499:dbl)
        n245 = Multiply(x=w493, y=w505) -> (x*y=w498:dbl)
        n246 = Multiply(x=w513, y=w493) -> (x*y=w497:dbl)
        n247 = Multiply(x=w535, y=w493) -> (x*y=w496:dbl)
        n248 = Divide(x=w513, y=9600.0) -> (x/y=w508:dbl)
        n249 = Divide(x=w505, y=9600.0) -> (x/y=w509:dbl)
        n250 = local read "start x"() -> (w506:dbl)
        n251 = local read "start y"() -> (w507:dbl)
        n252 = Add(x=w508, y=w506) -> (x+y=→"x position 2":dbl)
        n253 = Add(x=w509, y=w507) -> (x+y=→"y position 2":dbl)
        n254 = call "Wait3"("Count(mSec)"=u32 20) -> ("Tick Count(mSec)"=→"Tick Count(mSec) 2":u32)
      }
      n255 = call "Tick Count"() -> ("Tick Count(uSec)"=w205:u32)
      n256 = while {
        stop <- FALSE stop-if-true
        n257 = shared-variable "RT myRIO Target - Overlord\\Localization_Variables_r0.lvlib\\loc_x"() -> (w454:dbl)  [unwired: 1 in, 1 out]
        "loc_x" <- w454
        n258 = shared-variable "RT myRIO Target - Overlord\\Localization_Variables_r0.lvlib\\loc_y"() -> (→"loc_y":dbl)  [unwired: 1 in, 1 out]
        n259 = shared-variable "RT myRIO Target - Overlord\\Localization_Variables_r0.lvlib\\loc_theta"() -> (→"loc_theta":dbl)  [unwired: 1 in, 1 out]
        n260 = local read "x goal"() -> (w453:dbl)
        n261 = Subtract(x=w454, y=w453) -> (x-y=→"distance to goal":dbl)
      }
      n262 = while {
        tunnel: w204 -> [w583]
        stop <- FALSE stop-if-true
        # "left mid"
        n263 = xnode "Read/Write Control"("FPGA VI Reference In"=w583) -> ("SYS.SELECTA"=→"SYS.SELECTA":u8)  [unwired: 1 in, 2 out]
        n264 = xnode "Read/Write Control"("FPGA VI Reference In"=w583) -> ("ENC.A_a.CNTR"=→"ENC.A_a.CNTR":u32, "ENC.A_b.CNTR"=→"ENC.A_b.CNTR":u32, "ENC.A_c.CNTR"=→"ENC.A_c.CNTR":u32, "ENC.B_a.CNTR"=→"ENC.B_a.CNTR":u32, "ENC.B_b.CNTR"=→"ENC.B_b.CNTR":u32, "ENC.B_c.CNTR"=→"ENC.B_c.CNTR":u32)  [unwired: 1 in, 2 out]
        n265 = Wait (ms)(milliseconds to wait=u32 20) -> ()  [unwired: 1 out]
        n266 = case shown="True" "Encoder Reset" {
          tunnel: w583 -> [_ w594]
          frame False {
          }
          frame True {
            n267 = flat-sequence {
              tunnel: w594 -> [w599]
              tunnel: [w597] -> w596
              tunnel: w596 -> [w601]
              tunnel: [w601] -> w595
              tunnel: w595 -> [w604]
              tunnel: [w603] -> _
              frame #0 {
                w598 = u8 60 ("SYS.SELECTA")
                w600 = u8 3 ("ENC.B_c.CNFG")
                n268 = xnode "Read/Write Control"("FPGA VI Reference In"=w599, "ENC.A_a.CNFG"=w600, "ENC.A_b.CNFG"=w600, "ENC.A_c.CNFG"=w600, "ENC.B_a.CNFG"=w600, "ENC.B_b.CNFG"=w600, "ENC.B_c.CNFG"=w600, "SYS.SELECTA"=w598, "SYS.SELECTB"=w598) -> ("FPGA VI Reference Out"=w597:refnum<k20>)  [unwired: 1 in, 1 out]
              }
              frame #1 {
                n269 = Wait (ms)(milliseconds to wait=u32 10) -> ()  [unwired: 1 out]
              }
              frame #2 {
                w605 = u8 1 ("ENC.B_c.CNFG")
                n270 = xnode "Read/Write Control"("FPGA VI Reference In"=w604, "ENC.A_a.CNFG"=w605, "ENC.A_b.CNFG"=w605, "ENC.A_c.CNFG"=w605, "ENC.B_a.CNFG"=w605, "ENC.B_b.CNFG"=w605, "ENC.B_c.CNFG"=w605) -> ("FPGA VI Reference Out"=w603:refnum<k20>)  [unwired: 1 in, 1 out]
              }
            }
          }
        }
      }
      n271 = while {
        tunnel: w201 -> [w485]
        tunnel: [w486] -> _
        tunnel: w200 -> [w473]
        shift-right: [w472] -> _
        shift-left: _ -> [w481]
        shift-right: ["pid reset left"] -> _
        shift-left: _ -> [w464]
        tunnel: [w473] -> _
        tunnel: w197 -> [w475]
        tunnel: w196 -> [w474]
        stop <- "pid reset left" stop-if-true
        # "*****\n\n(true is supposed\nto be 0)"
        n272 = local read "left setpoint"() -> (w471:dbl)
        n273 = local read "stop motors"() -> (w476:dbl)
        n274 = local read "encoder stop switch"() -> (w468:dbl)
        n275 = Multiply(x=w476, y=w471) -> (x*y=w470:dbl)
        n276 = Add(x=0.5, y=w471) -> (x+y=→"desired pwm left":dbl)
        n277 = call "Elapsed Time2"("Reset"=w464) -> ("Elapsed Time (s)"=w463:dbl, "Time has Elapsed"=w467:bool)  [unwired: 11 in, 6 out]
        "Elapsed Time (s) Left" <- w463
        n278 = Multiply(x=w470, y=w468) -> (x*y=w469:dbl)
        n279 = local read "scale"() -> (w457:dbl)
        n280 = Multiply(x=w457, y=w469) -> (x*y=w458:dbl)
        n281 = Not(x=w467) -> (.not. x?=w480:bool)
        ".not. x? 3" <- w480
        n282 = Greater Or Equal?(x=w463, y=4.0) -> (x >= y?=w461:bool)
        n283 = case shown="True" w461 {
          tunnel: [1.0 1.0] -> w465
          frame False {
          }
          frame True {
          }
        }
        n284 = Multiply(x=w458, y=w465) -> (x*y=w466:dbl)
        n285 = call-poly <vilib>:"PID.vi"("reinitialize? (F)"=w480, "output range"="output range left", "PID gains"="PID gains left", "process variable"=w481, "setpoint"=w466) -> ("dt out (s)"=→"dt out (s) left":dbl, "output"=w472:dbl)  [unwired: 5 in]
        n286 = Add(x=0.5, y=w472) -> (x+y=w459:dbl)
        "left wheels actual pwm" <- w459
        "left pwm" <- w459
        n287 = call <vilib>:"Set Duty Cycle and Frequency.vi"("Frequency [Hz]"=w473, "Duty Cycle"=w459, "PWM Ref In"=w485) -> ("PWM Ref Out"=w486:T7)  [unwired: 6 in, 1 out]
        n288 = call <vilib>:"Set Duty Cycle and Frequency.vi"("Frequency [Hz]"=w473, "Duty Cycle"=w459, "PWM Ref In"=w475) -> ()  [unwired: 6 in, 2 out]
        n289 = call <vilib>:"Set Duty Cycle and Frequency.vi"("Frequency [Hz]"=w473, "Duty Cycle"=w459, "PWM Ref In"=w474) -> ()  [unwired: 6 in, 2 out]
        "PID feedback Left" <- w481
      }
      n290 = while {
        tunnel: w202 -> [w579]
        tunnel: [w580] -> _
        tunnel: [w567] -> _
        shift-right: [w566] -> _
        shift-left: _ -> [w575]
        shift-right: ["pid reset right"] -> _
        shift-left: _ -> [w559]
        tunnel: w200 -> [w567]
        tunnel: w199 -> [w569]
        tunnel: w198 -> [w568]
        stop <- "pid reset right" stop-if-true
        w553 = 0.5
        # "******"
        n291 = local read "right setpoint"() -> (w565:dbl)
        n292 = local read "scale"() -> (w570:dbl)
        n293 = Multiply(x=w570, y=w565) -> (x*y=w564:dbl)
        n294 = local read "encoder stop switch"() -> (w562:dbl)
        n295 = Add(x=0.5, y=w564) -> (x+y=→"desired pwm right":dbl)
        n296 = call "Elapsed Time"("Reset"=w559) -> ("Elapsed Time (s)"=w558:dbl, "Time has Elapsed"=w556:bool)  [unwired: 11 in, 6 out]
        "Elapsed Time (s) Right" <- w558
        n297 = local read "stop motors"() -> (w551:dbl)
        n298 = Multiply(x=w564, y=w562) -> (x*y=w563:dbl)
        n299 = Multiply(x=w551, y=w563) -> (x*y=w552:dbl)
        n300 = Not(x=w556) -> (.not. x?=w574:bool)
        ".not. x? 2" <- w574
        n301 = Greater Or Equal?(x=w558, y=4.0) -> (x >= y?=w555:bool)
        n302 = case shown="True" w555 {
          tunnel: [1.0 1.0] -> w560
          frame False {
          }
          frame True {
          }
        }
        n303 = Multiply(x=w552, y=w560) -> (x*y=w561:dbl)
        n304 = call-poly <vilib>:"PID.vi"("reinitialize? (F)"=w574, "output range"="output range right", "PID gains"="PID gains right", "process variable"=w575, "setpoint"=w561) -> ("dt out (s)"=→"dt out (s) right":dbl, "output"=w566:dbl)  [unwired: 5 in]
        n305 = Add(x=w553, y=w566) -> (x+y=→"right wheels actual pwm" →"right pwm":dbl)
        n306 = call <vilib>:"Set Duty Cycle and Frequency.vi"("Frequency [Hz]"=w567, "Duty Cycle"=w553, "PWM Ref In"=w568) -> ()  [unwired: 6 in, 2 out]
        n307 = call <vilib>:"Set Duty Cycle and Frequency.vi"("Frequency [Hz]"=w567, "Duty Cycle"=w553, "PWM Ref In"=w569) -> ()  [unwired: 6 in, 2 out]
        n308 = call <vilib>:"Set Duty Cycle and Frequency.vi"("Frequency [Hz]"=w567, "Duty Cycle"=w553, "PWM Ref In"=w579) -> ("PWM Ref Out"=w580:T7)  [unwired: 6 in, 1 out]
        "PID feedback Right" <- w575
      }
      n309 = while {
        shift-right: [w624] -> _
        shift-left: _ -> [w623]
        shift-right: [w621] -> _
        shift-left: w205 -> [w620]
        tunnel: w203 -> [w631]
        stop <- FALSE stop-if-true
        n310 = xnode "Read/Write Control"("FPGA VI Reference In"=w631) -> ("ENC.A_a.CNTR"=w630:u32, "ENC.A_b.CNTR"=w629:u32, "ENC.A_c.CNTR"=w628:u32, "ENC.B_a.CNTR"=w627:u32, "ENC.B_b.CNTR"=w626:u32, "ENC.B_c.CNTR"=w625:u32)  [unwired: 1 in, 2 out]
        n311 = call "Wait"("Count(mSec)"=u32 20) -> ()  [unwired: 1 out]
        n312 = Build Array(w630, w629, w628, w627, w626, w625) -> (w624:u32[])
        n313 = Subtract(x=w624, y=w623) -> (x-y=w622:u32[])
        n314 = call "Tick Count2"() -> ("Tick Count(uSec)"=w621:u32)
        n315 = Index Array(array=w622) -> (element #1=w619:u32, element #2=w618:u32, element #3=w617:u32, element #4=w616:u32, element #5=w615:u32, element #6=w614:u32)  [unwired: 6 in]
        n316 = Subtract(x=w621, y=w620) -> (x-y=w613:u32)
        n317 = call "Encoder-Velocity_Conversion (SubVI).vi"("delta  Encoder Count"=w618, "dt (uSec)"=w613) -> ("Rotational Velocity (RPS)"=w608:dbl)  [unwired: 7 in, 2 out]
        "LM Rot Velocity (rot/s)" <- w608
        n318 = call "Encoder-Velocity_Conversion (SubVI).vi"("delta  Encoder Count"=w617, "dt (uSec)"=w613) -> ("Rotational Velocity (RPS)"=w607:dbl)  [unwired: 7 in, 2 out]
        "LF Rot Velocity (rot/s)" <- w607
        n319 = call "Encoder-Velocity_Conversion (SubVI).vi"("delta  Encoder Count"=w619, "dt (uSec)"=w613) -> ("Rotational Velocity (RPS)"=w609:dbl)  [unwired: 7 in, 2 out]
        "LR Rot Velocity (rot/s)" <- w609
        n320 = call "Encoder-Velocity_Conversion (SubVI).vi"("delta  Encoder Count"=w616, "dt (uSec)"=w613) -> ("Rotational Velocity (RPS)"=w606:dbl)  [unwired: 7 in, 2 out]
        "RR Rot Velocity (rot/s)" <- w606
        n321 = call "Encoder-Velocity_Conversion (SubVI).vi"("delta  Encoder Count"=w615, "dt (uSec)"=w613) -> ("Rotational Velocity (RPS)"=w610:dbl)  [unwired: 7 in, 2 out]
        "RM Linear Velocity (rot/s)" <- w610
        n322 = call "Encoder-Velocity_Conversion (SubVI).vi"("delta  Encoder Count"=w614, "dt (uSec)"=w613) -> ("Rotational Velocity (RPS)"=w611:dbl)  [unwired: 7 in, 2 out]
        "RF Linear Velocity (rot/s)" <- w611
        n323 = Bundle("Rotational Velocity (RPS)"=w609, "Rotational Velocity (RPS)"=w608, "Rotational Velocity (RPS)"=w607, "Rotational Velocity (RPS)"=w606, "Rotational Velocity (RPS)"=w610, "Rotational Velocity (RPS)"=w611) -> (→"Current Rot Velocity (rot/s)":T4)  [unwired: 1 in]
      }
      n324 = while {
        stop <- FALSE stop-if-true
        # "(current-start)/(goal-start)"
        n325 = shared-variable "RT myRIO Target - Overlord\\Localization_Variables_r0.lvlib\\loc_x"() -> (w222:dbl)  [unwired: 1 in, 1 out]
        n326 = In Range and Coerce(upper limit=50.0, x=w222, lower limit=-50.0) -> (In Range?=w223:bool)  [unwired: 1 out]
        n327 = case shown="False" w223 {
          tunnel: w222 -> [w242 _]
          frame False {
            n328 = Greater?(x=w242, y=5.0) -> (0:w240:bool)
            n329 = case shown="True" w240 {
              frame False {
                n330 = local write "right setpoint"(0.133) -> ()
                n331 = local write "left setpoint"(0.1) -> ()
              }
              frame True {
                n332 = local write "right setpoint"(0.1) -> ()
                n333 = local write "left setpoint"(0.1333) -> ()
              }
            }
          }
          frame True {
            "right setpoint" <- 0.05
            "left setpoint" <- 0.05
          }
        }
        n334 = shared-variable "RT myRIO Target - Overlord\\Localization_Variables_r0.lvlib\\loc_x"() -> (w206:dbl)  [unwired: 1 in, 1 out]
        n335 = local read "start x"() -> (w207:dbl)
        n336 = Subtract(x=w207, y="x goal") -> (x-y=w208:dbl)
        n337 = Subtract(x=w206, y=w207) -> (x-y=w211:dbl)
        n338 = Subtract(x="x goal", y=w207) -> (x-y=w210:dbl)
        n339 = Sign(1:w208) -> (0:w213:dbl)
        n340 = Divide(x=w211, y=w210) -> (x/y=w214:dbl)
        "percent away from x goal" <- w214
        n341 = local read "Encoder Reset"() -> (w221:bool)
        n342 = Greater?(x=w214, y=0.75) -> (0:w215:bool)
        n343 = Not(x="motor killswitch") -> (.not. x?=w219:bool)
        n344 = Boolean To (0,1)(Boolean=w219) -> (0, 1=w217:i16)
        n345 = case shown="True" w215 {
          tunnel: w214 -> [_ w232]
          tunnel: w213 -> [w227 w229]
          frame False {
            n346 = Multiply(x=1.0, y=w227) -> (x*y=→"scale":dbl)
          }
          frame True {
            n347 = Greater?(x=w232, y=1.0) -> (0:w230:bool)
            n348 = case shown="True" w230 {
              tunnel: w229 -> [w235 _]
              frame False {
                n349 = Multiply(x=w235, y=0.85) -> (x*y=w233:dbl)
                n350 = local write "scale"(w233) -> ()
              }
              frame True {
                n351 = local write "scale"(0.0) -> ()
                "goal reached" <- TRUE
              }
            }
          }
        }
        n352 = case shown="False" w221 {
          tunnel: [w238 w239] -> w220
          frame False {
            w238 = 1.0
            n353 = local write "reset x y 2"(w238) -> ()
          }
          frame True {
            w239 = 0.0
            n354 = local write "reset x y 2"(w239) -> ()
            "reset x y 2" <- w239
          }
        }
        "encoder stop switch" <- w220
        n355 = local write "stop motors"(w217) -> ()
      }
    }
  }
